vi "open_gcode_exe.vi"() -> ()   [LabVIEW 2018]
panel:
  in  "wait until completion?":bool
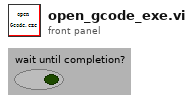
[diagram p1: front panel]
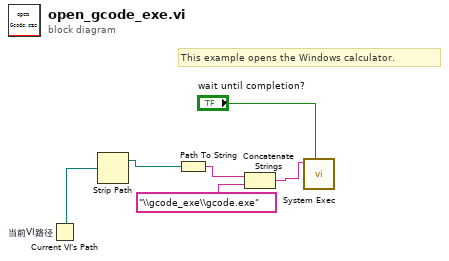
[diagram p0: block diagram]
diagram:
  # "This example opens the Windows calculator."
  n1 = Current VI's Path "当前VI路径"() -> (path=w5:path)
  n2 = Strip Path(path=w5) -> (stripped path=w2:path)  [unwired: 1 out]
  n3 = Path To String(path=w2) -> (string=w4:string)
  n4 = Concatenate Strings(w4, "\\gcode_exe\\gcode.exe") -> (w1:string)
  n5 = call <vilib>:"System Exec.vi"("wait until completion? (T)"="wait until completion?", "command line"=w1) -> ()  [unwired: 6 in, 4 out]
